vi "Update.vi"(8 "error in (no error)":errorcluster, 11 "PongBall in":refnum<class "PongBall.lvclass">) -> (0 "error out":errorcluster, 3 "PongBall out":refnum<class "PongBall.lvclass">)   [LabVIEW 2019, in "RT_Game.lvlib" / "PongBall.lvclass"]
uses:
  PongBall.lvclass
  C:/Users/FreshBob/Dropbox/VIs/myRIO_GameConsole/RT/RT_Game/GameObject/GameObject.lvclass
  Velocity.ctl
  GameObject/GameObject.lvclass/GameObject.ctl
  PongBall.lvclass/PongBall.ctl
  GameObject/Read position.vi
  GameObject/Read size.vi
  Globals.vi
  RT_Sprite/RT_Sprite.lvclass
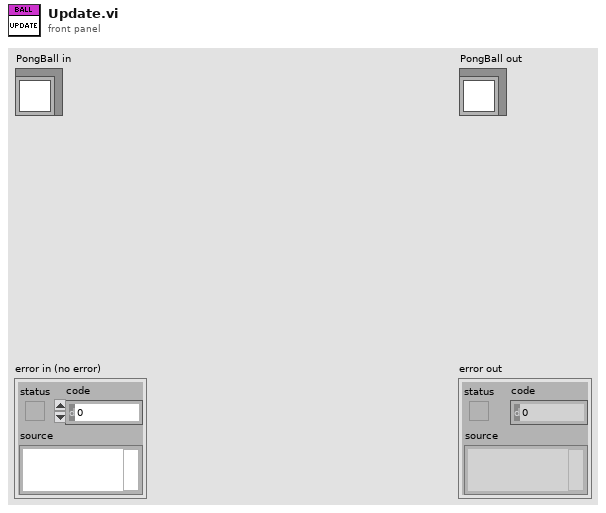
[diagram p1: front panel]
types:
  T1 = typedef "Velocity.ctl" = cluster{"x":dbl, "y":dbl}
  T2 = typedef "RT_Game.lvlib/Game.lvclass/Coordinate.ctl" = cluster{"x":dbl, "y":dbl}
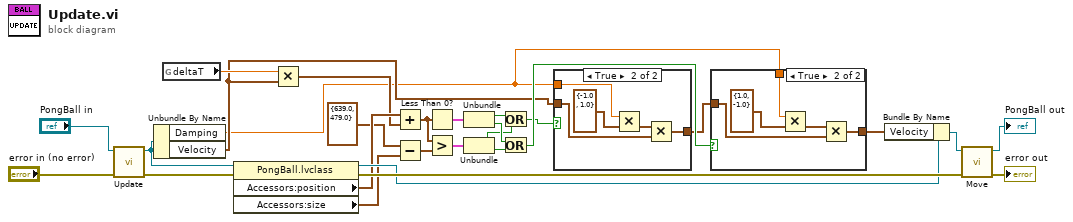
[diagram p0: block diagram]
diagram:
  n1 = call-parent "Update.vi"("error in (no error)"="error in (no error)", "GameObject in"="PongBall in") -> ("error out"=w15:errorcluster, "GameObject out"=w16:refnum<class "PongBall.lvclass">)  [unwired: 8 in]
  n2 = Unbundle By Name(w16) -> ("Damping"=w1:dbl, "Velocity"=w3:T1)
  n3 = global read "Globals.vi" "deltaT"() -> (w10:dbl)
  n4 = property class="PongBall.lvclass"(reference=w16, error in=w15) -> (reference out=w25:refnum<class "PongBall.lvclass">, error out=w26:errorcluster, "Accessors:position"=w24:T2, "Accessors:size"=w8:T2)
  n5 = Multiply(x=w10, y=w3) -> (x*y=w11:T1)
  n6 = Add(x=w24, y=w11) -> (x+y=w22:T2)
  n7 = Subtract(x=T1 {"x"=639.0, "y"=479.0} ("y"), y=w8) -> (x-y=w9:T1)
  n8 = Less Than 0?(x=w22) -> (x < 0?=w23:cluster{"x":bool, "y":bool})
  n9 = Greater?(x=w22, y=w9) -> (0:w20:cluster{"x":bool, "y":bool})
  n10 = Unbundle(w23) -> ("x"=w6:bool, "y"=w18:bool)
  n11 = Unbundle(w20) -> ("x"=w5:bool, "y"=w17:bool)
  n12 = Or(x=w6, y=w5) -> (x .or. y?=w4:bool)
  n13 = Or(x=w18, y=w17) -> (x .or. y?=w7:bool)
  n14 = case shown="True" w4 {
    tunnel: w3 -> [w29 w34]
    tunnel: [w29 w32] -> w2
    tunnel: w1 -> [_ w30]
    frame False {
    }
    frame True {
      n15 = Multiply(x=w30, y=T1 {"x"=-1.0, "y"=1.0} ("x")) -> (x*y=w31:T1)
      n16 = Multiply(x=w31, y=w34) -> (x*y=w32:T1)
    }
  }
  n17 = case shown="True" w7 {
    tunnel: w2 -> [w35 w40]
    tunnel: [w35 w38] -> w19
    tunnel: w1 -> [_ w36]
    frame False {
    }
    frame True {
      n18 = Multiply(x=w36, y=T1 {"x"=1.0, "y"=-1.0} ("x")) -> (x*y=w37:T1)
      n19 = Multiply(x=w37, y=w40) -> (x*y=w38:T1)
    }
  }
  n20 = Bundle By Name(cluster=w25, "Velocity"=w19) -> (w13:refnum<class "PongBall.lvclass">)
  n21 = call "Move.vi"("error in (no error)"=w26, "PongBall in"=w13) -> ("error out"=→"error out":errorcluster, "PongBall out"=→"PongBall out":refnum<class "PongBall.lvclass">)  [unwired: 8 in]
